vi "Write Pole.vi"(1 "Fehler (Eingang)":errorcluster, 2 "array":string[](array[string]), 3 "Port for write head":refnum<visa-resource-name>="COM4", 4 "Port for Powersupply":refnum<visa-resource-name>="COM3") -> (0 "Fehler (Ausgang)":errorcluster)   [LabVIEW 2013]
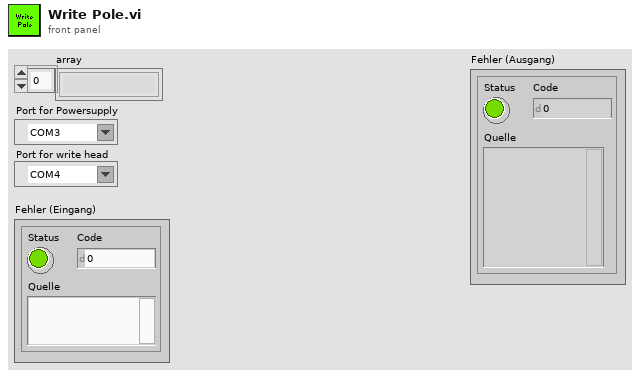
[diagram p1: front panel]
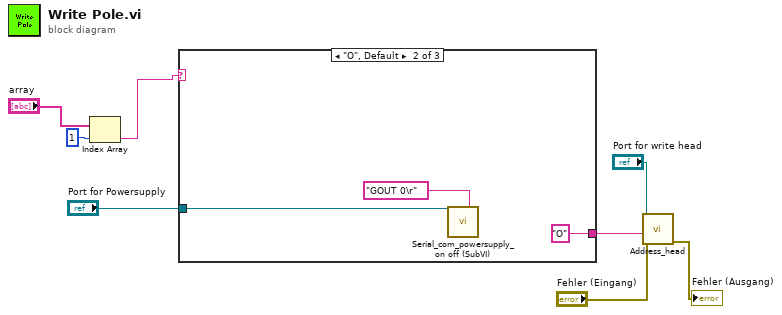
[diagram p0: block diagram]
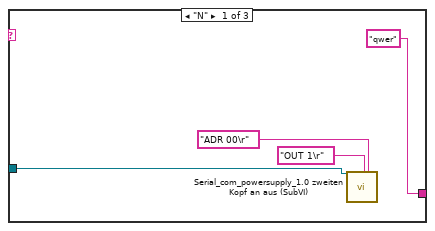
[diagram p2: hidden frame]
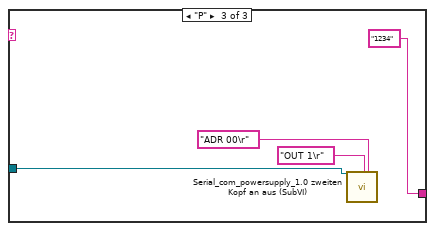
[diagram p3: hidden frame]
diagram:
  n1 = Index Array(array="array", index=1) -> (element=w6:string)
  n2 = case shown="\"O\", Default" w6 {
    tunnel: "Port for Powersupply" -> [w10 w14 w19]
    tunnel: ["qwer" "O" "1234"] -> w4
    frame "N" {
      n3 = call "Serial_com_powersupply_1.0 zweiten Kopf an aus (SubVI).vi"("VISA-Referenz (Eingang)"=w10, "string to write 3"="OUT 1\r", "string to write"="ADR 00\r") -> ()  [unwired: 22 in, 3 out]
    }
    frame "O", Default {
      n4 = call "Serial_com_powersupply_on off (SubVI).vi"("VISA-Referenz (Eingang)"=w14, "string to write"="GOUT 0\r") -> ()  [unwired: 25 in, 1 out]
    }
    frame "P" {
      n5 = call "Serial_com_powersupply_1.0 zweiten Kopf an aus (SubVI).vi"("VISA-Referenz (Eingang)"=w19, "string to write 3"="OUT 1\r", "string to write"="ADR 00\r") -> ()  [unwired: 22 in, 3 out]
    }
  }
  n6 = call "Address_head.vi"("Fehler (Eingang)"="Fehler (Eingang)", "Write"=w4, "VISA-Ressourcenname"="Port for write head") -> ("Fehler (Ausgang)"=→"Fehler (Ausgang)":errorcluster)  [unwired: 5 in, 2 out]
